vi "5.两种表格控件不覆盖.vi"() -> ()   [LabVIEW 2018]
panel:
  out "表格控件 2":string[][](table)
  out "表格控件缓冲区 2":string[][](array[string])
  out "表格控件缓冲区1":string[][](array[string])
  out "表格控件1":string[][](table)
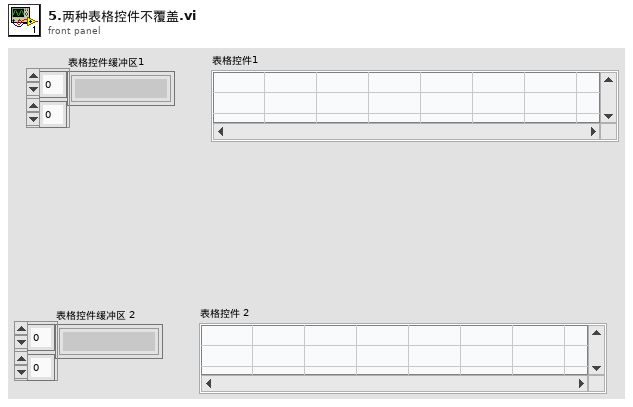
[diagram p1: front panel]
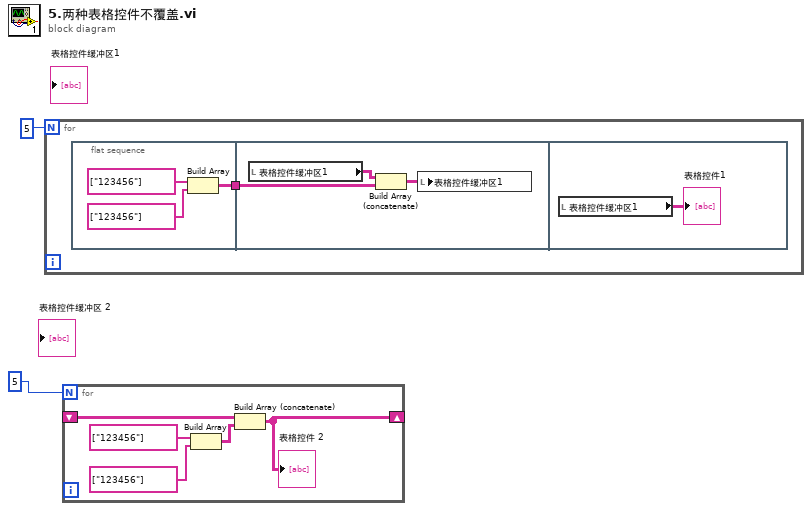
[diagram p0: block diagram]
diagram:
  n1 = for {
    N: 5 -> [_]
    n2 = flat-sequence {
      tunnel: [w4] -> w3
      tunnel: w3 -> [w8]
      frame #0 {
        n3 = Build Array(string[] ["123456"], string[] ["123456"]) -> (w4:string[][])
      }
      frame #1 {
        n4 = local read "表格控件缓冲区1"() -> (w9:string[][])
        n5 = Build Array (concatenate)(w9, w8) -> (w7:string[][])
        n6 = local write "表格控件缓冲区1"(w7) -> ()
      }
      frame #2 {
        n7 = local read "表格控件缓冲区1"() -> (→"表格控件1":string[][])
      }
    }
  }
  n8 = for {
    N: 5 -> [_]
    shift-right: [w11] -> _
    shift-left: _ -> [w12]
    n9 = Build Array(string[] ["123456"], string[] ["123456"]) -> (w15:string[][])
    n10 = Build Array (concatenate)(w12, w15) -> (w11:string[][])
    "表格控件 2" <- w11
  }
